vi "Create All Message Queues.vi"(8 "error in (no error)":errorcluster) -> (0 "error out":errorcluster, 3 "Message Queues out":T1)   [LabVIEW 2025]
doc: "This VI creates and initializes all the message queues for your application. If your application requires more than one message queue, right-click the \"Message Queues\" constant above and select Open Type Def. Add the new Message Queue(s) to the type definition, then initialize them in this VI."
uses:
  LABVIEW_QCM_v2.0/Labview_code/QCM_2.0_LV_1.2/QMH/Message Queue/All Message Queues.ctl
  LABVIEW_QCM_v2.0/Labview_code/QCM_2.0_LV_1.2/QMH/Message Queue/Message Cluster.ctl
  LABVIEW_QCM_v2.0/Labview_code/QCM_2.0_LV_1.2/QMH/Message Queue/Enqueue Message (Single).vi
  LABVIEW_QCM_v2.0/Labview_code/QCM_2.0_LV_1.2/QMH/Message Queue/Message Queue.lvlib
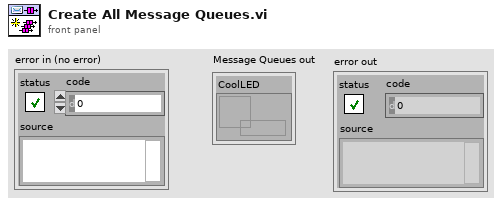
[diagram p1: front panel]
types:
  T1 = typedef "Message Queue.lvlib/All Message Queues.ctl" = cluster{"CoolLED":refnum<queue>}
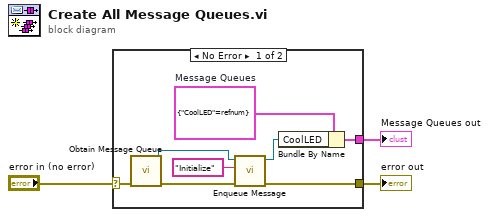
[diagram p0: block diagram]
diagram:
  n1 = case shown="No Error" "error in (no error)" {
    selector: "error in (no error)" -> [w6 w12]
    tunnel: [w11 w12] -> w3
    tunnel: [w10 _] -> w2
    frame No Error {
      w7 = T1 {"CoolLED"=refnum}  # Message Queues
      n2 = call "Obtain Message Queue.vi"("error in (no error)"=w6) -> ("error out"=w9:errorcluster, "Message Queue"=w4:refnum<queue>)  [unwired: 9 in]
      n3 = call-poly "Enqueue Message.vi"("error in (no error)"=w9, "Message"="Initialize", "Message Queue"=w4) -> ("error out"=w11:errorcluster, "dup Message Queue"=w5:refnum<queue>)  [unwired: 7 in]
      n4 = Bundle By Name(cluster=w7, "CoolLED"=w5) -> (w10:T1)
    }
    frame Error {
    }
  }
  "Message Queues out" <- w2
  "error out" <- w3
